vi "Data Edge Trigger 8 Samples.vi"(9 "Trigger Level":i16, 10 "Newer Data In":u64, 11 "Older Data In":u64) -> (3 "Trigger":bool)   [LabVIEW 2020]
doc: "This VI looks at the data from the NI 5771 to determine if a Data Edge trigger has happened given the Trigger Level."
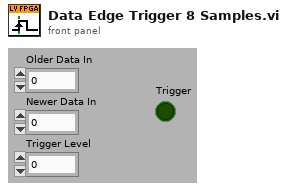
[diagram p1: front panel]
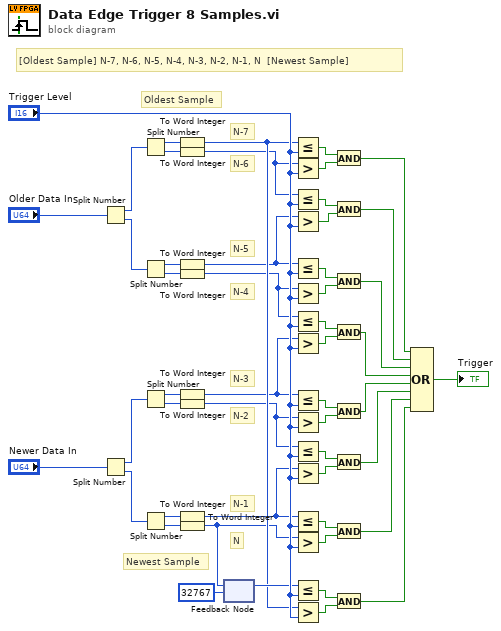
[diagram p0: block diagram]
diagram:
  # "[Oldest Sample] N-7, N-6, N-5, N-4, N-3, N-2, N-1, N  [Newest Sample]"
  # "N"
  # "N-1"
  # "N-2"
  # "N-3"
  # "N-4"
  # "N-5"
  # "N-6"
  # "N-7"
  # "Oldest Sample"
  # "Newest Sample"
  n1 = Split Number(x="Older Data In") -> (hi(x)=w50:u32, lo(x)=w49:u32)
  n2 = Split Number(x="Newer Data In") -> (hi(x)=w48:u32, lo(x)=w47:u32)
  n3 = Split Number(x=w50) -> (hi(x)=w11:u16, lo(x)=w19:u16)
  n4 = Split Number(x=w49) -> (hi(x)=w18:u16, lo(x)=w17:u16)
  n5 = Split Number(x=w48) -> (hi(x)=w16:u16, lo(x)=w15:u16)
  n6 = Split Number(x=w47) -> (hi(x)=w14:u16, lo(x)=w13:u16)
  n7 = To Word Integer(number=w11) -> (16bit integer=w8:i16)
  n8 = To Word Integer(number=w19) -> (16bit integer=w7:i16)
  n9 = To Word Integer(number=w18) -> (16bit integer=w6:i16)
  n10 = To Word Integer(number=w17) -> (16bit integer=w5:i16)
  n11 = To Word Integer(number=w16) -> (16bit integer=w4:i16)
  n12 = To Word Integer(number=w15) -> (16bit integer=w3:i16)
  n13 = To Word Integer(number=w14) -> (16bit integer=w2:i16)
  n14 = To Word Integer(number=w13) -> (16bit integer=w1:i16)
  n15 = feedback #1(i16 32767) -> (w12:i16)
  n16 = feedback-in #1(w1) -> ()
  n17 = Less Or Equal?(x=w8, y="Trigger Level") -> (x <= y?=w45:bool)
  n18 = Greater?(x=w7, y="Trigger Level") -> (0:w46:bool)
  n19 = Less Or Equal?(x=w7, y="Trigger Level") -> (x <= y?=w44:bool)
  n20 = Greater?(x=w6, y="Trigger Level") -> (0:w43:bool)
  n21 = Less Or Equal?(x=w6, y="Trigger Level") -> (x <= y?=w38:bool)
  n22 = Greater?(x=w5, y="Trigger Level") -> (0:w37:bool)
  n23 = Less Or Equal?(x=w5, y="Trigger Level") -> (x <= y?=w39:bool)
  n24 = Greater?(x=w4, y="Trigger Level") -> (0:w40:bool)
  n25 = Less Or Equal?(x=w4, y="Trigger Level") -> (x <= y?=w35:bool)
  n26 = Greater?(x=w3, y="Trigger Level") -> (0:w36:bool)
  n27 = Less Or Equal?(x=w3, y="Trigger Level") -> (x <= y?=w34:bool)
  n28 = Greater?(x=w2, y="Trigger Level") -> (0:w33:bool)
  n29 = Less Or Equal?(x=w2, y="Trigger Level") -> (x <= y?=w30:bool)
  n30 = Greater?(x=w1, y="Trigger Level") -> (0:w29:bool)
  n31 = Less Or Equal?(x=w12, y="Trigger Level") -> (x <= y?=w31:bool)
  n32 = Greater?(x=w8, y="Trigger Level") -> (0:w32:bool)
  n33 = And(x=w45, y=w46) -> (x .and. y?=w42:bool)
  n34 = And(x=w44, y=w43) -> (x .and. y?=w41:bool)
  n35 = And(x=w38, y=w37) -> (x .and. y?=w28:bool)
  n36 = And(x=w39, y=w40) -> (x .and. y?=w27:bool)
  n37 = And(x=w35, y=w36) -> (x .and. y?=w26:bool)
  n38 = And(x=w34, y=w33) -> (x .and. y?=w25:bool)
  n39 = And(x=w30, y=w29) -> (x .and. y?=w24:bool)
  n40 = And(x=w31, y=w32) -> (x .and. y?=w23:bool)
  n41 = Compound Arithmetic op=OR(w42, w41, w28, w27, w26, w25, w24, w23) -> (→"Trigger":bool)
